vi "new attach communicator message.vi"(11 "comm":refnum<class "communicator.lvclass">) -> (2 "ID":string, 3 "message":refnum<class "communicator message.lvclass">)   [LabVIEW 2015, in "queue manager.lvclass"]
uses:
  queue manager.lvclass
  message/communicator message.lvclass
  communicator/communicator.lvclass
  new communicator message.ctl
  communicator/communicator.lvclass/communicator.ctl
  message/communicator message.lvclass/communicator message.ctl
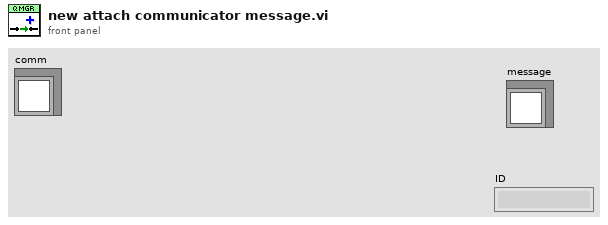
[diagram p1: front panel]
types:
  T1 = typedef "queue manager.lvclass/new communicator message.ctl" = cluster{"ID":string, "comm":refnum<class "communicator.lvclass">}
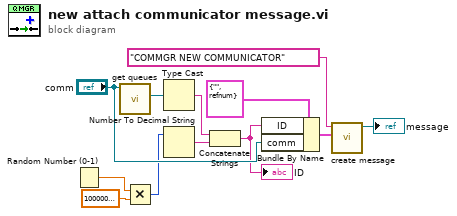
[diagram p0: block diagram]
diagram:
  n1 = Random Number (0-1)() -> (number: 0 to 1=w6:dbl)
  n2 = call "get queues.vi"("communicator in"="comm") -> ("to worker"=w8:refnum<queue>)  [unwired: 9 in, 1 out]
  n3 = Multiply(x=w6, y=1000000000000000.0) -> (x*y=w4:u64)
  n4 = Type Cast(x=w8) -> (*(type *) &x=w7:string)  [unwired: 1 in]
  n5 = Number To Decimal String(number=w4) -> (decimal integer string=w3:string)  [unwired: 1 in]
  n6 = Concatenate Strings(w7, w3) -> (w2:string)
  "ID" <- w2
  n7 = Bundle By Name(cluster=T1 {"ID"="", "comm"=refnum} ("new comm message"), "ID"=w2, "comm"="comm") -> (w1:T1)
  n8 = call "create message.vi"("data"=w1, "ID"="COMMGR NEW COMMUNICATOR") -> ("message"=→"message":refnum<class "communicator message.lvclass">)  [unwired: 9 in]
